vi "adjoint.vi"(1 "3x3 matrix":dbl[][](array[numeric])) -> (0 "Adjoint of matrix":dbl[][](array[numeric]))   [LabVIEW 2015]
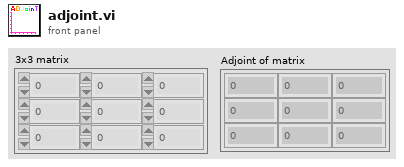
[diagram p1: front panel]
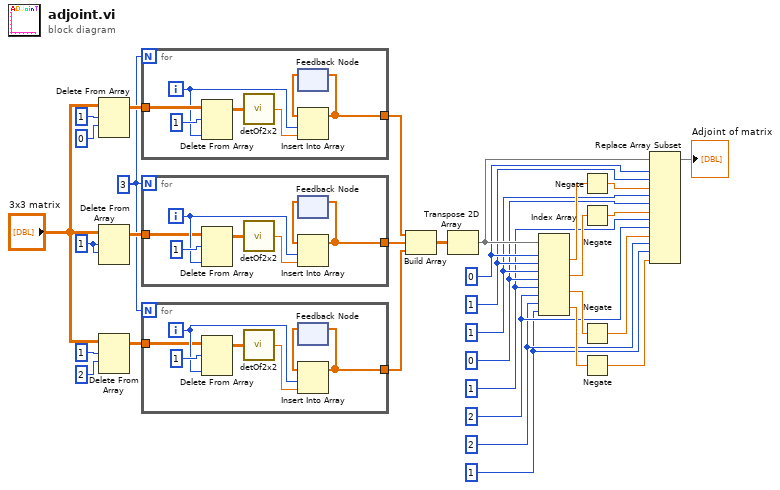
[diagram p0: block diagram]
diagram:
  w2 = 1 ("disabled index (col)")
  w3 = 2 ("index (row)")
  w6 = 2 ("disabled index (col)")
  w7 = 1 ("index (row)")
  w9 = 0 ("disabled index (col)")
  w10 = 1 ("index (row)")
  w11 = 1 ("disabled index (col)")
  w12 = 0 ("index (row)")
  w28 = 1 ("length")
  w27 = 3
  n1 = Delete From Array(array="3x3 matrix", length=1, index (row)=0) -> (array with subset deleted=w30:dbl[][])  [unwired: 1 in, 1 out]
  n2 = Delete From Array(array="3x3 matrix", length=w28, index (row)=w28) -> (array with subset deleted=w29:dbl[][])  [unwired: 1 in, 1 out]
  n3 = Delete From Array(array="3x3 matrix", length=1, index (row)=2) -> (array with subset deleted=w24:dbl[][])  [unwired: 1 in, 1 out]
  n4 = for {
    N: w27 -> [_]
    tunnel: w30 -> [w39]
    tunnel: [w33] -> w22
    i -> [w35]
    n5 = Delete From Array(array=w39, length=1, index (col)=w35) -> (array with subset deleted=w37:dbl[][])  [unwired: 1 in, 1 out]
    n6 = call "detOf2x2.vi"("2x2Matrix"=w37) -> ("Determinant"=w34:dbl)
    n7 = feedback #1() -> (w36:dbl[])  [unwired: 1 in]
    n8 = Insert Into Array(array=w36, index=w35, new element=w34) -> (w33:dbl[])
    n9 = feedback-in #1(w33) -> ()
  }
  n10 = for {
    N: w27 -> [_]
    tunnel: w29 -> [w41]
    tunnel: [w40] -> w21
    i -> [w43]
    n11 = Delete From Array(array=w41, length=1, index (col)=w43) -> (array with subset deleted=w45:dbl[][])  [unwired: 1 in, 1 out]
    n12 = call "detOf2x2.vi"("2x2Matrix"=w45) -> ("Determinant"=w42:dbl)
    n13 = feedback #2() -> (w44:dbl[])  [unwired: 1 in]
    n14 = Insert Into Array(array=w44, index=w43, new element=w42) -> (w40:dbl[])
    n15 = feedback-in #2(w40) -> ()
  }
  n16 = for {
    N: w27 -> [_]
    tunnel: w24 -> [w48]
    tunnel: [w47] -> w20
    i -> [w50]
    n17 = Delete From Array(array=w48, length=1, index (col)=w50) -> (array with subset deleted=w52:dbl[][])  [unwired: 1 in, 1 out]
    n18 = call "detOf2x2.vi"("2x2Matrix"=w52) -> ("Determinant"=w49:dbl)
    n19 = feedback #3() -> (w51:dbl[])  [unwired: 1 in]
    n20 = Insert Into Array(array=w51, index=w50, new element=w49) -> (w47:dbl[])
    n21 = feedback-in #3(w47) -> ()
  }
  n22 = Build Array(w22, w21, w20) -> (w19:dbl[][])
  n23 = Transpose 2D Array(2D array=w19) -> (transposed array=w18:dbl[][])
  n24 = Index Array(array=w18, index (row) #1=w12, index (col) #1=w11, index (row) #2=w10, index (col) #2=w9, index (row) #3=w7, index (col) #3=w6, index (row) #4=w3, index (col) #4=w2) -> (element #1=w17:dbl, element #2=w16:dbl, element #3=w15:dbl, element #4=w14:dbl)
  n25 = Negate(x=w17) -> (-x=w13:dbl)
  n26 = Negate(x=w16) -> (-x=w8:dbl)
  n27 = Negate(x=w15) -> (-x=w5:dbl)
  n28 = Negate(x=w14) -> (-x=w4:dbl)
  n29 = Replace Array Subset(array=w18, new element #1=w13, index (row) #1=w12, index (col) #1=w11, new element #2=w8, index (row) #2=w10, index (col) #2=w9, new element #3=w5, index (row) #3=w7, index (col) #3=w6, new element #4=w4, index (row) #4=w3, index (col) #4=w2) -> (→"Adjoint of matrix":dbl[][])
